vi "TEST_SCRIPT.vi"() -> ()   [LabVIEW 2014]
panel:
  out "Byte2":u8 format="%.0x"
  out "Byte1":u8 format="%.0x"
  in  "Byte1 2":u8 format="%.0x"
  in  "Byte1":u8 format="%.0x"
  out "DAC Val":u16 format="%.0x"
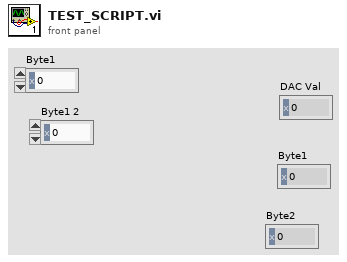
[diagram p1: front panel]
types:
  T1 = cluster{"Boolean array[0]":bool, "Boolean array[1]":bool, "Boolean array[2]":bool, "Boolean array[3]":bool, "Boolean array[4]":bool, "Boolean array[5]":bool, "Boolean array[6]":bool, "Boolean array[7]":bool}
  T2 = cluster{"unsigned byte array[0]":u8, "unsigned byte array[1]":u8, "unsigned byte array[2]":u8, "unsigned byte array[3]":u8, "unsigned byte array[4]":u8, "unsigned byte array[5]":u8, "unsigned byte array[6]":u8, "unsigned byte array[7]":u8, "unsigned byte array[8]":u8}
  T3 = cluster{"Boolean array[0]":bool, "Boolean array[1]":bool, "Boolean array[2]":bool, "Boolean array[3]":bool, "Boolean array[4]":bool, "Boolean array[5]":bool, "Boolean array[6]":bool, "Boolean array[7]":bool, "Boolean array[0]":bool, "Boolean array[1]":bool, "Boolean array[2]":bool, "Boolean array[3]":bool}
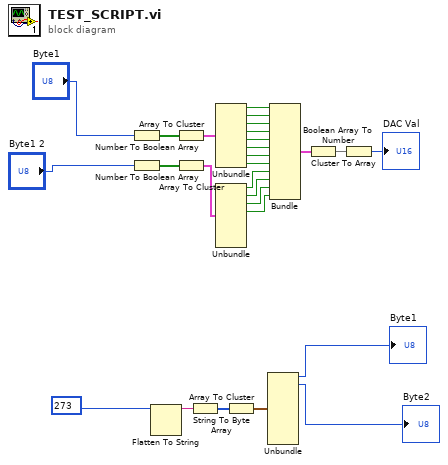
[diagram p0: block diagram]
diagram:
  n1 = Number To Boolean Array(number="Byte1") -> (Boolean array=w26:bool[])
  n2 = Number To Boolean Array(number="Byte1 2") -> (Boolean array=w24:bool[])
  n3 = Flatten To String(anything=u16 273) -> (data string=w4:string)  [unwired: 3 in, 2 out]
  n4 = Array To Cluster(array=w26) -> (cluster=w27:T1)
  n5 = Array To Cluster(array=w24) -> (cluster=w25:T1)
  n6 = String To Byte Array(string=w4) -> (unsigned byte array=w5:u8[])
  n7 = Unbundle(w27) -> ("Boolean array[0]"=w23:bool, "Boolean array[1]"=w22:bool, "Boolean array[2]"=w21:bool, "Boolean array[3]"=w20:bool, "Boolean array[4]"=w19:bool, "Boolean array[5]"=w18:bool, "Boolean array[6]"=w17:bool, "Boolean array[7]"=w16:bool)
  n8 = Unbundle(w25) -> ("Boolean array[0]"=w15:bool, "Boolean array[1]"=w14:bool, "Boolean array[2]"=w13:bool, "Boolean array[3]"=w12:bool)  [unwired: 4 out]
  n9 = Array To Cluster(array=w5) -> (cluster=w6:T2)
  n10 = Unbundle(w6) -> ("unsigned byte array[0]"=→"Byte1":u8, "unsigned byte array[1]"=→"Byte2":u8)  [unwired: 7 out]
  n11 = Bundle("Boolean array[0]"=w23, "Boolean array[1]"=w22, "Boolean array[2]"=w21, "Boolean array[3]"=w20, "Boolean array[4]"=w19, "Boolean array[5]"=w18, "Boolean array[6]"=w17, "Boolean array[7]"=w16, "Boolean array[0]"=w15, "Boolean array[1]"=w14, "Boolean array[2]"=w13, "Boolean array[3]"=w12) -> (w11:T3)  [unwired: 1 in]
  n12 = Cluster To Array(cluster=w11) -> (array=w10:bool[])
  n13 = Boolean Array To Number(Boolean array=w10) -> (number=→"DAC Val":u32)
